vi "DHT12 Get Temperature.vi"(1 "Data":u8[](array[numeric])) -> (0 "Temperature":dbl)   [LabVIEW 2020, in "lv_dht12.lvlib"]
uses:
  <vilib>/miidas/lv_dht12/lv_dht12.lvlib
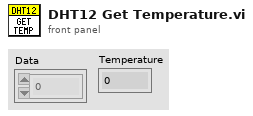
[diagram p1: front panel]
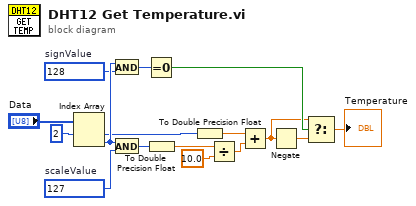
[diagram p0: block diagram]
diagram:
  w14 = u8 128  # signValue
  w15 = u8 127  # scaleValue
  n1 = Index Array(array="Data", index #1=2 ("index")) -> (element #1=w8:u8, element #2=w16:u8)  [unwired: 1 in]
  n2 = And(x=w16, y=w14) -> (x .and. y?=w7:u8)
  n3 = And(x=w16, y=w15) -> (x .and. y?=w13:u8)
  n4 = Equal To 0?(x=w7) -> (x = 0?=w6:bool)
  n5 = To Double Precision Float(number=w13) -> (double precision float=w12:dbl)
  n6 = To Double Precision Float(number=w8) -> (double precision float=w9:dbl)
  n7 = Divide(x=w12, y=10.0) -> (x/y=w10:dbl)
  n8 = Add(x=w9, y=w10) -> (x+y=w4:dbl)
  n9 = Negate(x=w4) -> (-x=w5:dbl)
  n10 = Select(t=w4, s=w6, f=w5) -> (s? t:f=→"Temperature":dbl)
